vi "Joystick to Data.vi"(1 "Rotation":dbl format="%#_13g", 2 "Joystick Y":dbl format="%#_13g", 3 "Joystick X":dbl format="%#_13g") -> (0 "Motor Commands":T1)   [LabVIEW 2018]
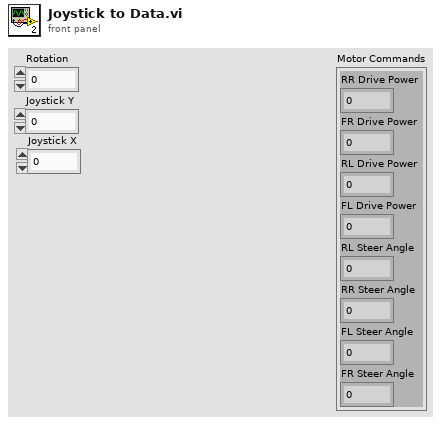
[diagram p1: front panel]
types:
  T1 = cluster{"RR Drive Power":dbl, "FR Drive Power":dbl, "RL Drive Power":dbl, "FL Drive Power":dbl, "RL Steer Angle":dbl, "RR Steer Angle":dbl, "FL Steer Angle":dbl, "FR Steer Angle":dbl}
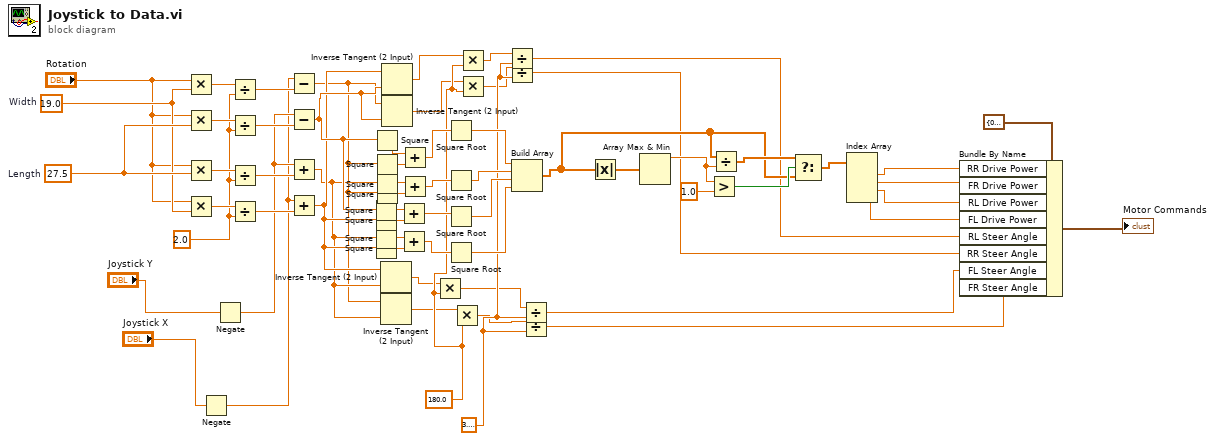
[diagram p0: block diagram]
diagram:
  w20 = 3.141592653589793
  w25 = 180.0
  w57 = 2.0
  w63 = 27.5  # Length
  w62 = 19.0  # Width
  n1 = Multiply(x="Rotation", y=w62) -> (x*y=w61:dbl)
  n2 = Multiply(x="Rotation", y=w63) -> (x*y=w60:dbl)
  n3 = Multiply(x="Rotation", y=w63) -> (x*y=w59:dbl)
  n4 = Multiply(x="Rotation", y=w62) -> (x*y=w58:dbl)
  n5 = Negate(x="Joystick X") -> (-x=w6:dbl)
  n6 = Negate(x="Joystick Y") -> (-x=w7:dbl)
  n7 = Divide(x=w61, y=w57) -> (x/y=w56:dbl)
  n8 = Divide(x=w60, y=w57) -> (x/y=w55:dbl)
  n9 = Divide(x=w59, y=w57) -> (x/y=w54:dbl)
  n10 = Divide(x=w58, y=w57) -> (x/y=w53:dbl)
  n11 = Subtract(x=w6, y=w56) -> (x-y=w41:dbl)
  n12 = Subtract(x=w7, y=w55) -> (x-y=w46:dbl)
  n13 = Add(x=w7, y=w54) -> (x+y=w42:dbl)
  n14 = Add(x=w6, y=w53) -> (x+y=w43:dbl)
  n15 = Square(x=w46) -> (x^2=w47:dbl)
  n16 = Square(x=w43) -> (x^2=w48:dbl)
  n17 = Square(x=w42) -> (x^2=w44:dbl)
  n18 = Square(x=w43) -> (x^2=w45:dbl)
  n19 = Square(x=w46) -> (x^2=w51:dbl)
  n20 = Square(x=w41) -> (x^2=w52:dbl)
  n21 = Square(x=w42) -> (x^2=w49:dbl)
  n22 = Square(x=w41) -> (x^2=w50:dbl)
  n23 = Inverse Tangent (2 Input)(1:w42, 2:w43) -> (0:w22:dbl)
  n24 = Inverse Tangent (2 Input)(1:w42, 2:w41) -> (0:w21:dbl)
  n25 = Inverse Tangent (2 Input)(1:w46, 2:w43) -> (0:w24:dbl)
  n26 = Inverse Tangent (2 Input)(1:w46, 2:w41) -> (0:w23:dbl)
  n27 = Add(x=w47, y=w48) -> (x+y=w39:dbl)
  n28 = Add(x=w44, y=w45) -> (x+y=w40:dbl)
  n29 = Add(x=w51, y=w52) -> (x+y=w37:dbl)
  n30 = Add(x=w49, y=w50) -> (x+y=w38:dbl)
  n31 = Multiply(x=w22, y=w25) -> (x*y=w17:dbl)
  n32 = Square Root(x=w37) -> (sqrt(x)=w33:dbl)
  n33 = Square Root(x=w38) -> (sqrt(x)=w34:dbl)
  n34 = Square Root(x=w39) -> (sqrt(x)=w35:dbl)
  n35 = Square Root(x=w40) -> (sqrt(x)=w36:dbl)
  n36 = Multiply(x=w21, y=w25) -> (x*y=w16:dbl)
  n37 = Multiply(x=w24, y=w25) -> (x*y=w19:dbl)
  n38 = Multiply(x=w23, y=w25) -> (x*y=w18:dbl)
  n39 = Divide(x=w19, y=w20) -> (x/y=w14:dbl)
  n40 = Divide(x=w18, y=w20) -> (x/y=w13:dbl)
  n41 = Build Array(w33, w34, w35, w36) -> (w27:dbl[])
  n42 = Divide(x=w17, y=w20) -> (x/y=w12:dbl)
  n43 = Divide(x=w16, y=w20) -> (x/y=w11:dbl)
  n44 = Absolute Value(x=w27) -> (abs(x)=w32:dbl[])
  n45 = Array Max & Min(array=w32) -> (max value=w30:dbl)  [unwired: 3 out]
  n46 = Greater?(x=w30, y=1.0) -> (0:w28:bool)
  n47 = Divide(x=w27, y=w30) -> (x/y=w29:dbl[])
  n48 = Select(t=w29, s=w28, f=w27) -> (s? t:f=w26:dbl[])
  n49 = Index Array(array=w26) -> (element #1=w4:dbl, element #2=w3:dbl, element #3=w2:dbl, element #4=w1:dbl)  [unwired: 4 in]
  n50 = Bundle By Name(cluster=T1 {"RR Drive Power"=0.0, "FR Drive Power"=0.0, "RL Drive Power"=0.0, "FL Drive Power"=0.0, "RL Steer Angle"=0.0, "RR Steer Angle"=0.0, "FL Steer Angle"=0.0, "FR Steer Angle"=0.0}, "RR Drive Power"=w4, "FR Drive Power"=w3, "RL Drive Power"=w2, "FL Drive Power"=w1, "RL Steer Angle"=w14, "RR Steer Angle"=w13, "FL Steer Angle"=w12, "FR Steer Angle"=w11) -> (→"Motor Commands":T1)
